vi "Read Options.vi"(1 "ZXing Options in":refnum<class "ZXing Options.lvclass">) -> (0 "Options":T1)   [LabVIEW 2020, in "feature_detection.lvlib" / "ZXing Options.lvclass"]
uses:
  ZXing Options.lvclass
  ZXing Options.lvclass/ZXing Options.ctl
  Binarizer.ctl
  EAN Add-On Symbol.ctl
  Text Mode.ctl
  Character Set.ctl
  Format.ctl
  Options-Data.ctl
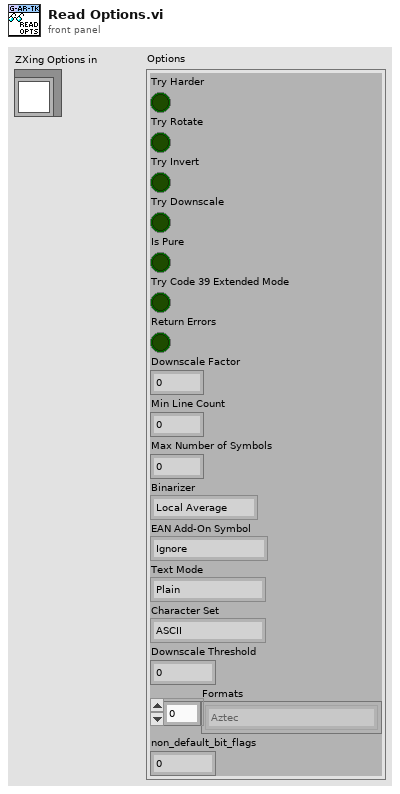
[diagram p1: front panel]
types:
  T1 = typedef "feature_detection.lvlib/ZXing Options.lvclass/Options-Data.ctl" = cluster{"Try Harder":bool, "Try Rotate":bool, "Try Invert":bool, "Try Downscale":bool, "Is Pure":bool, "Try Code 39 Extended Mode":bool, "Return Errors":bool, "Downscale Factor":u8, "Min Line Count":u8, "Max Number of Symbols":u8, "Binarizer":T2, "EAN Add-On Symbol":T3, "Text Mode":T4, "Character Set":T5, "Downscale Threshold":u16, "Formats":T6[], "non_default_bit_flags":u16}
  T2 = typedef "feature_detection.lvlib/ZXing Options.lvclass/Binarizer.ctl" = enum8{"Local Average", "Global Histogram", "Fixed Threshold", "Bool Cast"}
  T3 = typedef "feature_detection.lvlib/ZXing Options.lvclass/EAN Add-On Symbol.ctl" = enum8{"Ignore", "Read", "Require"}
  T4 = typedef "feature_detection.lvlib/ZXing Options.lvclass/Text Mode.ctl" = enum8{"Plain", "ECI", "HRI", "Hex", "Escaped"}
  T5 = typedef "feature_detection.lvlib/ZXing Options.lvclass/Character Set.ctl" = enum8{"ASCII", "ISO8859_1", "ISO8859_2", "ISO8859_3", "ISO8859_4", "ISO8859_5", "ISO8859_6", "ISO8859_7", "ISO8859_8", "ISO8859_9", "ISO8859_10", "ISO8859_11", "ISO8859_13", "ISO8859_14", "ISO8859_15", "ISO8859_16", "Cp437", "Cp1250", "Cp1251", "Cp1252", "Cp1256", "Shift_JIS", "Big5", "GB2312", "GB18030", "EUC_JP", "EUC_KR", "UTF16BE", "UTF8", "UTF16LE", "UTF32BE", "UTF32LE", "BINARY"}
  T6 = typedef "feature_detection.lvlib/ZXing Options.lvclass/Format.ctl" = enum8{"Aztec", "Codabar", "Code 39", "Code 93", "Code 128", "Data Bar", "Data Bar Expanded", "Data Matrix", "EAN 8", "EAN 13", "ITF", "Maxi Code", "PDF417", "QR Code", "UPCA", "UPCE", "Micro QR Code", "RM QR Code", "DX Film Edge", "Data Bar Limited"}
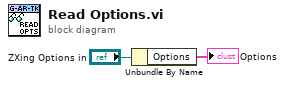
[diagram p0: block diagram]
diagram:
  n1 = Unbundle By Name("ZXing Options in") -> ("Options"=→"Options":T1)
